vi "Autonomous Independent.vi"() -> ()   [LabVIEW 2014]
doc: "This VI is called when autonomous begins, and will automatically be terminated when autonomous ends. You can carry out timed or sensor driven robot movement independently without needing to return to the caller."
uses:
  Robot Global Data.vi
panel:
  in  "Close Claw Power 4":dbl=-0.8
  in  "Elevator Power 4":dbl=-0.8
  in  "Elevator to Tote1 drop distance 4":dbl=50.0
  in  "open claw pwr 3":dbl=0.8
  in  "Close Claw Power 3":dbl=-0.8
  in  "Elevator Power 3":dbl=-0.8
  in  "Elevator to Tote1 drop distance 3":dbl=50.0
  in  "Elevator to drop to tote distance 3":dbl=50.0
  in  "Drop elevator pwr 3":dbl=-0.8
  in  "Move up to tote 3":dbl=50.0
  out "reach Tote? 3":bool
  in  "Elevator to Raise distance":dbl=50.0
  in  "Raise Elevator Power 3":dbl=0.8
  out "Current Step 2":string
  in  "Move up to auto zone 2":dbl
  out "reach auto zone? 2":bool
  in  "Left Set Point 2":dbl=-65.0
  in  "Right Set Point 2":dbl=-35.0
  out "Make Turn? 2":bool
  in  "open claw pwr 2":dbl=0.8
  in  "Wait Time between each step 2":dbl=0.5
  in  "Elevator to drop to tote distance 2":dbl=50.0
  in  "Drop elevator pwr 2":dbl=-0.8
  in  "Move up to tote 2":dbl=50.0
  out "reach Tote? 2":bool
  in  "Elevator to Raise RC above tote 2":dbl=50.0
  in  "Raise Elevator Power 2":dbl=0.8
  in  "Close Claw Power 2":dbl=-0.8
  in  "Elevator Power 2":dbl=-0.8
  in  "Elevator to Tote1 drop distance 2":dbl=50.0
  in  "Claw Open Power 2":dbl=0.8
  in  "close claw pwr":dbl=-0.8
  in  "Drop elevator pwr":dbl=-0.8
  in  "Open Claw Power":dbl=0.8
  in  "Raise Elevator Power":dbl=0.8
  in  "Close Claw Power":dbl=-0.8
  in  "Claw Open Power":dbl=-0.8
  in  "Move up to auto zone":dbl
  out "reach auto zone?":bool
  out "Make Turn?":bool
  in  "Right Set Point":dbl=-35.0
  in  "Left Set Point":dbl=-65.0
  in  "Elevator to drop to tote distance":dbl=50.0
  in  "Elevator to Raise RC above tote":dbl=50.0
  in  "Elevator to RC drop distance":dbl=50.0
  out "Reach Distance?":bool
  in  "Elevator Power":dbl=-0.8
  in  "Wait Time between each step":dbl=0.5
  out "Current Step":string
  out "Right Encoder":dbl
  out "Left Encoder":dbl
  in  "Go Staight Distance":dbl=-50.0
  out "reach Tote?":bool
  in  "Move up to tote":dbl=50.0
  in  "Left Range":cluster{"output high":dbl, "output low":dbl}={"output high"=0.75, "output low"=-0.75} {"output low" format="%.2f"; "output high" format="%.2f"}
  in  "Left Gains":T1={"proportional gain (Kc)"=0.25, "integral time (Ti, min)"=0.0, "derivative time (Td, min)"=0.0} {"derivative time (Td, min)" format="%.3f"; "integral time (Ti, min)" format="%.3f"; "proportional gain (Kc)" format="%.3f"}
  in  "Right Gains":T1={"proportional gain (Kc)"=0.25, "integral time (Ti, min)"=0.0, "derivative time (Td, min)"=0.0} {"derivative time (Td, min)" format="%.3f"; "integral time (Ti, min)" format="%.3f"; "proportional gain (Kc)" format="%.3f"}
  in  "Right Range":cluster{"output high":dbl, "output low":dbl}={"output high"=0.75, "output low"=-0.75} {"output low" format="%.2f"; "output high" format="%.2f"}
  # "Auton Options"
  # "Be sure to right-click and choose Data Operations>>Make Current Value default if you want to save the array values with the VI"
  # "Stack RC on Tote and take them to auto zone"
  # "Stack RC on Tote and take them to auto zone"
  # "Open Claw"
  # "Open Claw"
  # "Drop Elevator to RC"
  # "Drop Elevator to Tote 1"
  # "Close Claw on RC"
  # "Close Claw on Tote 1"
  # "Raise RC above Tote"
  # "Raise Tote 1 above Tote 2"
  # "Approach Tote"
  # "Approach Tote 2"
  # "Lower tote 1 onto Tote 2"
  # "Open Claw"
  # "Open Claw"
  # "Drop Elevator to Tote"
  # "Close Claw on Tote"
  # "Drop Elevator to Tote 2"
  # "Turn Left"
  # "Close Claw on Tote 2"
  # "Go to Auto Zone"
  # "Raise Totes 1&2 above Tote 3"
  # "Approach Tote 3"
  # "Lower tote 1 & 2 onto Tote 3"
  # "Open Claw"
  # "Drop Elevator to Tote 3"
  # "Close Claw on Tote 3"
  # "Turn Right"
  # "Go to Auto Zone"
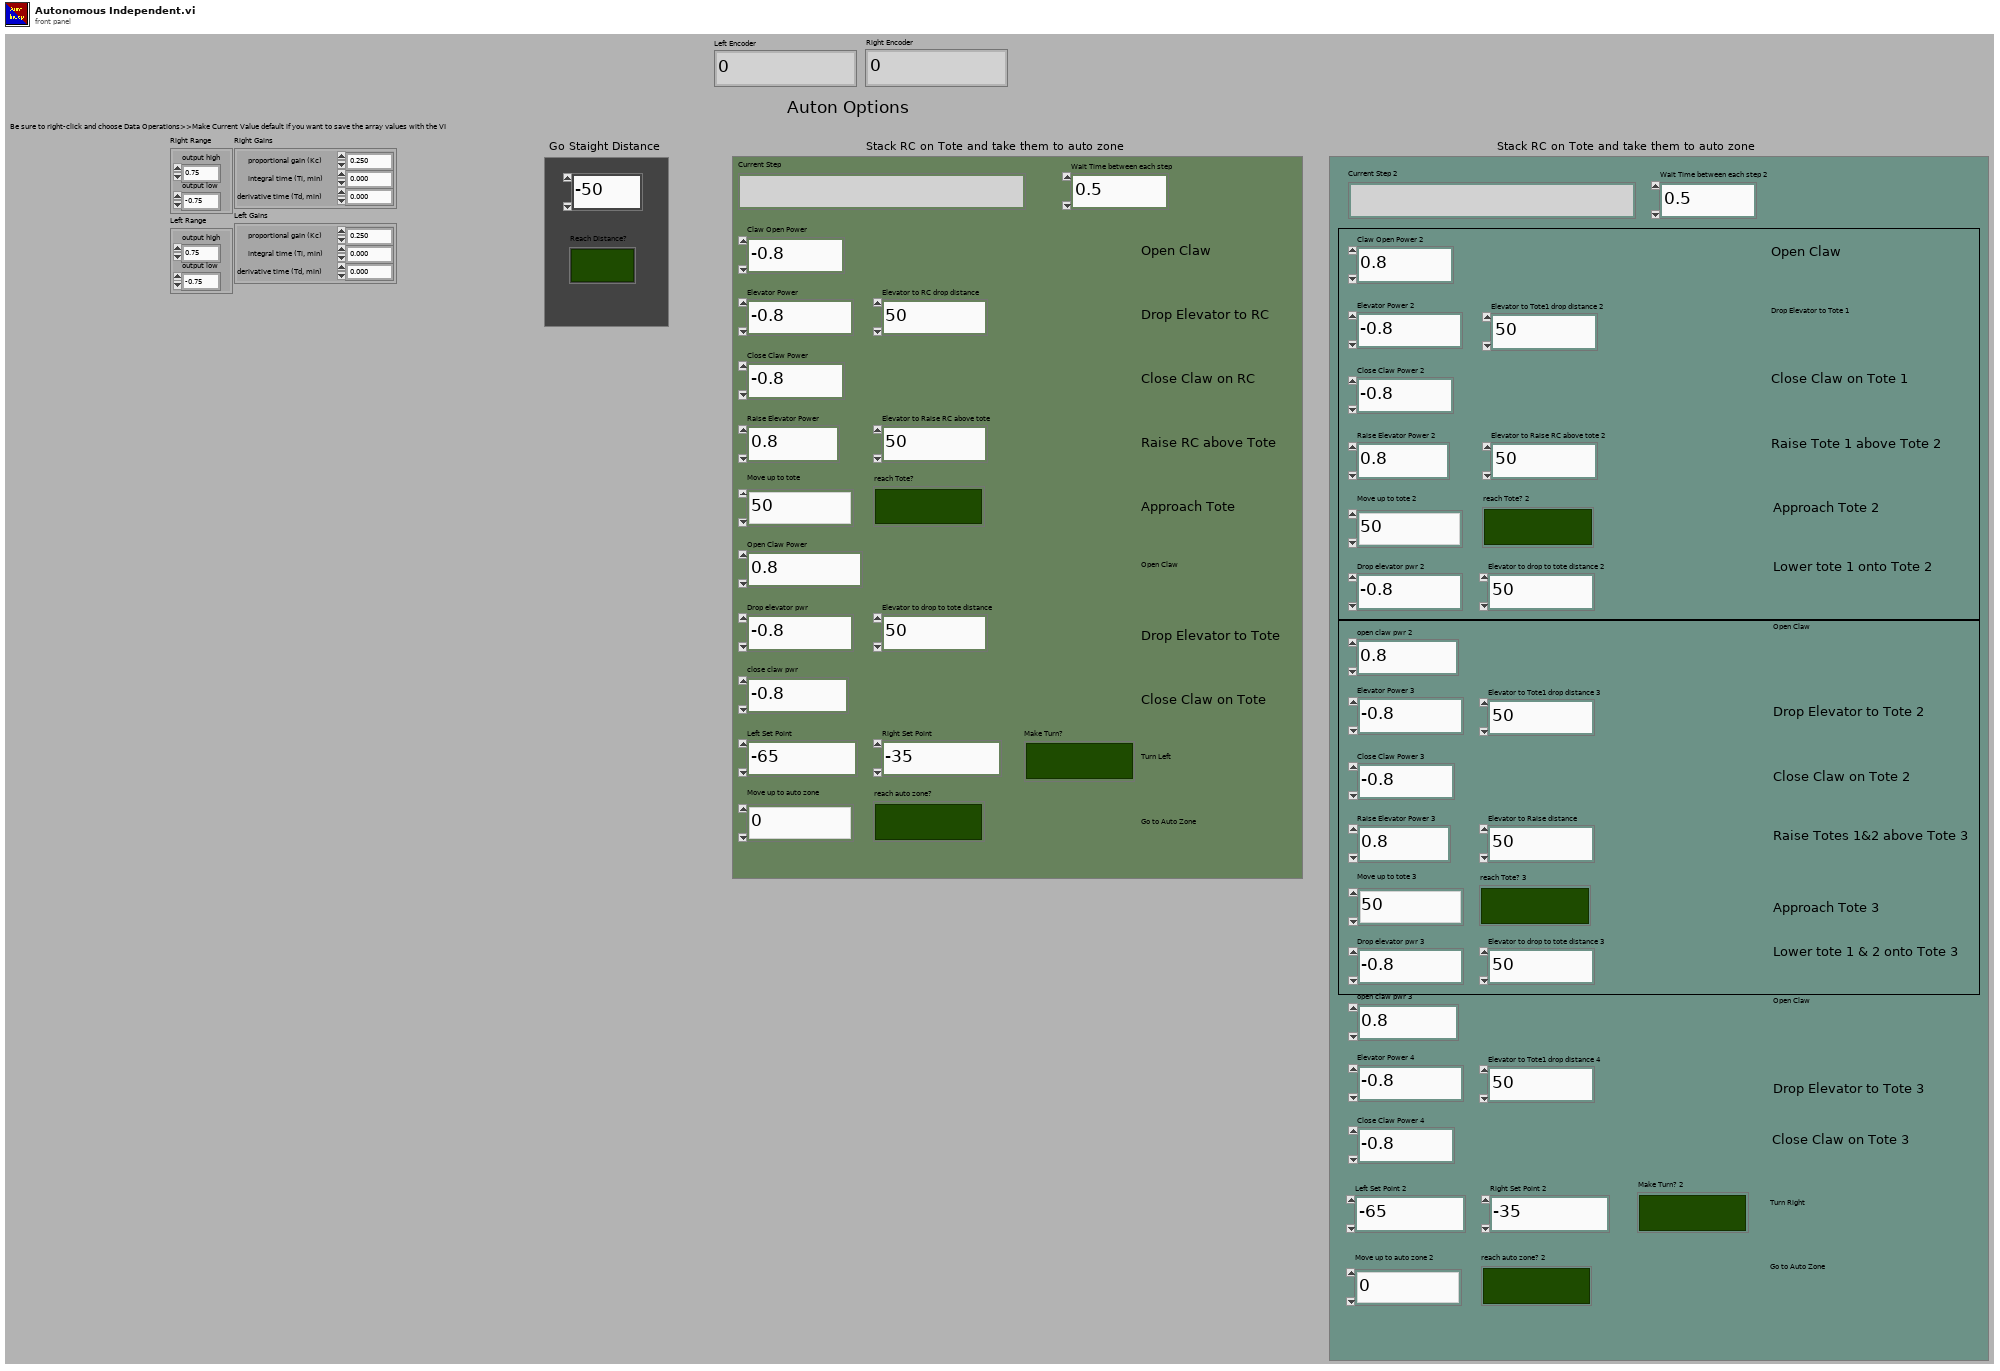
[diagram p1: front panel]
types:
  T1 = cluster{"proportional gain (Kc)":dbl, "integral time (Ti, min)":dbl, "derivative time (Td, min)":dbl}
  T2 = typedef "WPI_MotorControlDeviceRef.ctl" = cluster{"DeviceStatus":errorcluster, "Type":T3, "PWM":cluster{"Controller":T4, "PWM Channel":T5, "DeadBand":T6}, "CAN":cluster{"Device Number":u8, "Control Mode":T7, "Semaphore":T8, "Max Vout":dbl, "TalonSRX Control Mode":T9}, "Invert":bool, "TransformRef":T10, "InvTransformRef":T10}
  T3 = typedef "WPI_MotorControlType.ctl" = enum16{"PWM", "CAN", "CANTalonSRX"}
  T4 = typedef "FPGA_TypedefDigitalModule.ctl" = enum16{"Controller 1"}
  T5 = typedef "FPGA_DIOPWMChannel.ctl" = enum8{"PWM 0", "PWM 1", "PWM 2", "PWM 3", "PWM 4", "PWM 5", "PWM 6", "PWM 7", "PWM 8", "PWM 9", "PWM MXP 0", "PWM MXP 1", "PWM MXP 2", "PWM MXP 3", "PWM MXP 4", "PWM MXP 5", "PWM MXP 6", "PWM MXP 7", "PWM MXP 8", "PWM MXP 9", "Invalid"}
  T6 = typedef "WPI_PWMDeadband.ctl" = cluster{"Name":string, "maxPositivePwm":i32, "minPositivePwm":i32, "centerPwm":i32, "maxNegativePwm":i32, "minNegativePwm":i32, "angularRange":u16}
  T7 = typedef "WPI_CANJaguar_ControlMode.ctl" = enum8{"Percent VBus", "Current", "Speed", "Position", "Voltage"}
  T8 = typedef "Semaphore RefNum" = refnum<k1>
  T9 = typedef "WPI_CANTalonSRX_APIControlMode.ctl" = enum8{"Percent VBus", "Speed", "Position", "Slave", "Unchanged / Invalid"}
  T10 = typedef "WPI_PWMTransform_ConPane.ctl" = refnum<vi>
  T11 = typedef "WPI_EncoderDevRef.ctl" = cluster{"DevStatus":errorcluster, "EncoderIndex":T12, "CounterIndex":T13, "DistancePerCount":dbl, "Decoding Type":T14}
  T12 = typedef "FPGA_EncoderIdx.ctl" = enum8{"Enc 0", "Enc 1", "Enc 2", "Enc 3", "Enc 4", "Enc 5", "Enc 6", "Enc 7", "Invalid"}
  T13 = typedef "FPGA_CounterCtrSystemIndex.ctl" = enum8{"Ctr 0", "Ctr 1", "Ctr 2", "Ctr 3", "Ctr 4", "Ctr 5", "Ctr 6", "Ctr 7", "Invalid"}
  T14 = typedef "WPI_EncoderType.ctl" = enum16{"1x", "2x", "4x"}
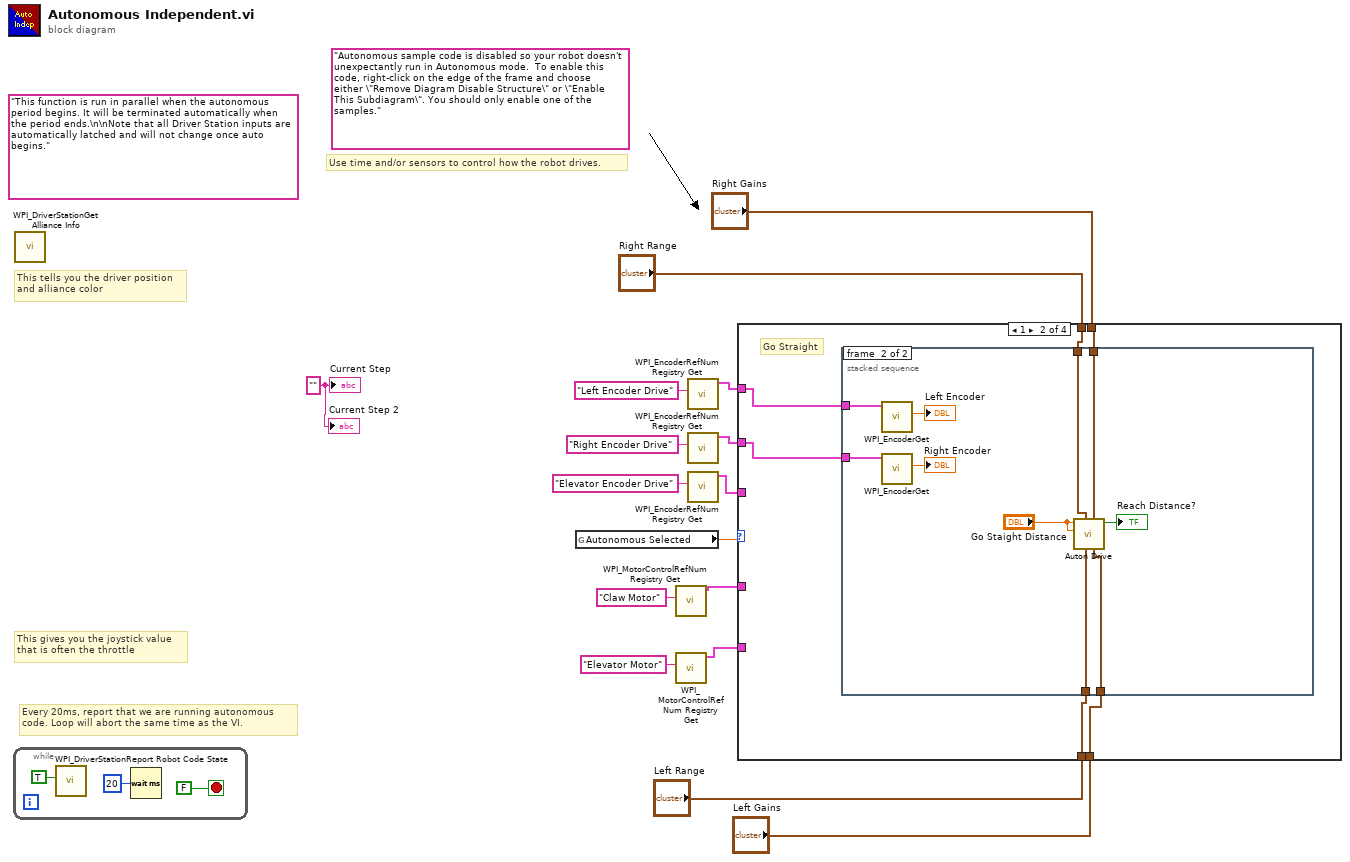
[diagram p0: block diagram]
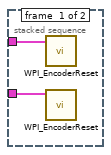
[diagram p3: hidden frame]
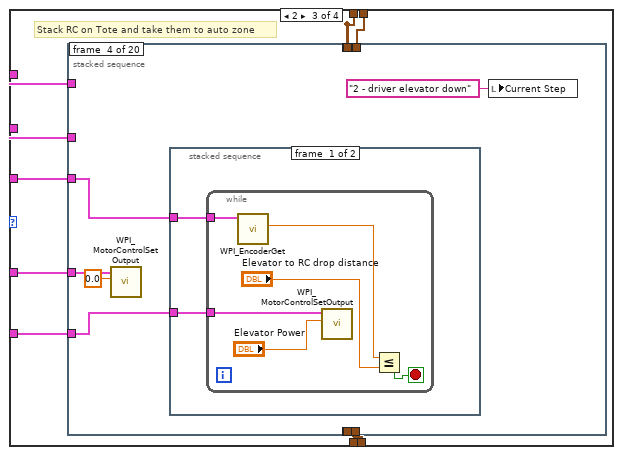
[diagram p4: hidden frame]
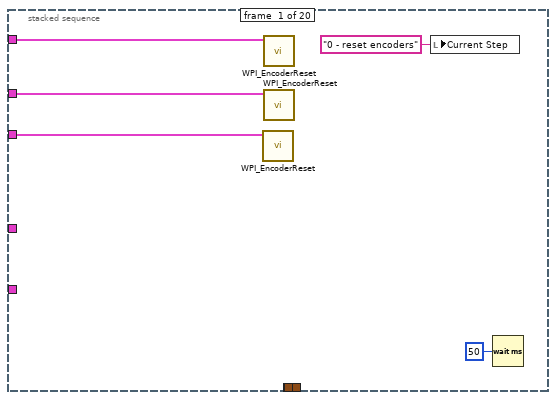
[diagram p5: hidden frame]
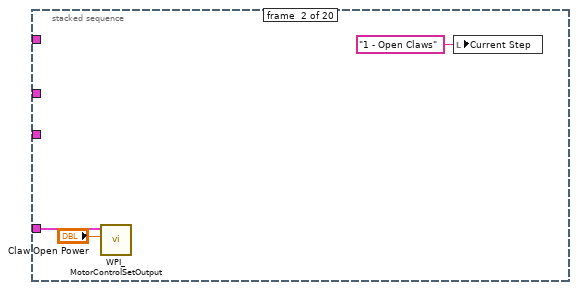
[diagram p6: hidden frame]
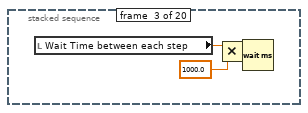
[diagram p7: hidden frame]
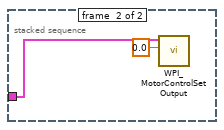
[diagram p8: hidden frame]
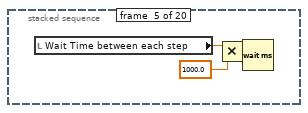
[diagram p9: hidden frame]
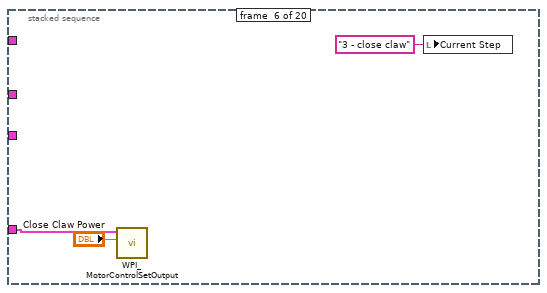
[diagram p10: hidden frame]
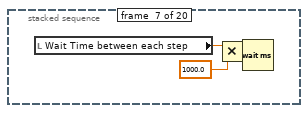
[diagram p11: hidden frame]
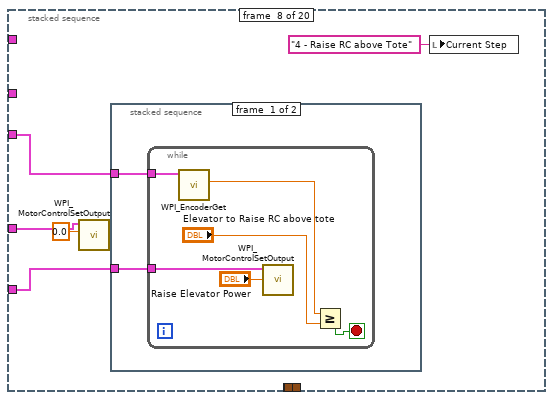
[diagram p12: hidden frame]
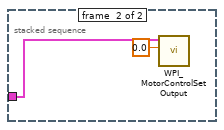
[diagram p13: hidden frame]
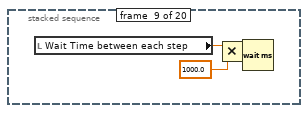
[diagram p14: hidden frame]
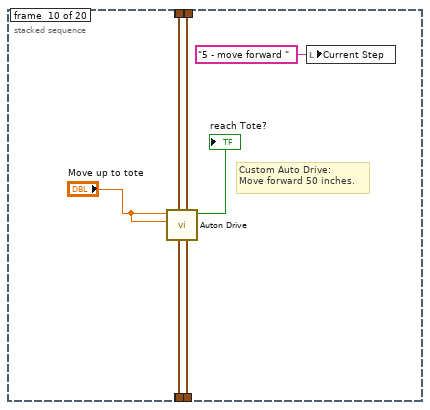
[diagram p15: hidden frame]
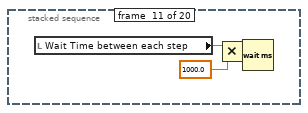
[diagram p16: hidden frame]
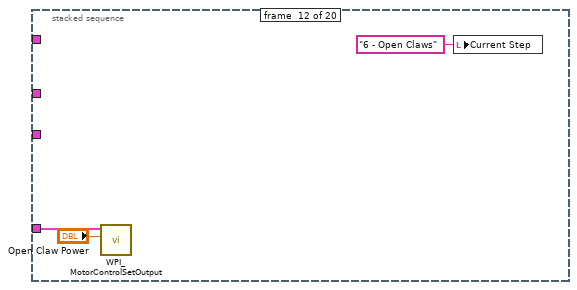
[diagram p17: hidden frame]
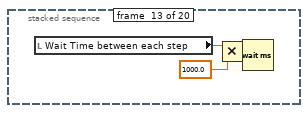
[diagram p18: hidden frame]
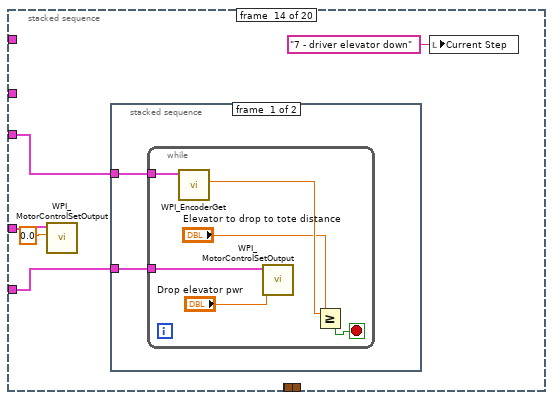
[diagram p19: hidden frame]
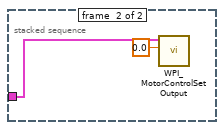
[diagram p20: hidden frame]
diagram:
  w1 = "" ("Current Step")
  (unwired) "Autonomous sample code is disabled so your robot doesn't unexpectantly run in Autonomous mode.  To enable this code, right-click on the edge of the frame and choose either \"Remove Diagram Disable Structure\" or \"Enable This Subdiagram\". You should only enable one of the samples."
  (unwired) "This function is run in parallel when the autonomous period begins. It will be terminated automatically when the period ends.\n\nNote that all Driver Station inputs are automatically latched and will not change once auto begins."
  # "Every 20ms, report that we are running autonomous\ncode. Loop will abort the same time as the VI."
  # "This gives you the joystick value\nthat is often the throttle"
  # "Use time and/or sensors to control how the robot drives."
  # "This tells you the driver position\nand alliance color"
  n1 = while {
    stop <- FALSE stop-if-true
    n2 = call <vilib>:"WPI_DriverStationReport Robot Code State.vi"("Autonomous"=TRUE) -> ()  [unwired: 10 in, 1 out]
    n3 = Wait (ms)(milliseconds to wait=u32 20) -> ()  [unwired: 1 out]
  }
  n4 = call <vilib>:"WPI_DriverStationGet Alliance Info.vi"() -> ()  [unwired: 12 out]
  n5 = global read "Robot Global Data.vi" "Autonomous Selected"() -> (w6:dbl)
  n6 = call <vilib>:"WPI_MotorControlRefNum Registry Get.vi"("refnum name"="Claw Motor") -> ("MotorControlDevRef"=w3:T2)  [unwired: 9 in, 1 out]
  n7 = call <vilib>:"WPI_MotorControlRefNum Registry Get.vi"("refnum name"="Elevator Motor") -> ("MotorControlDevRef"=w2:T2)  [unwired: 9 in, 1 out]
  n8 = call <vilib>:"WPI_EncoderRefNum Registry Get.vi"("refnum name"="Left Encoder Drive") -> ("EncoderDevRef"=w8:T11)  [unwired: 9 in, 1 out]
  n9 = call <vilib>:"WPI_EncoderRefNum Registry Get.vi"("refnum name"="Right Encoder Drive") -> ("EncoderDevRef"=w7:T11)  [unwired: 9 in, 1 out]
  n10 = call <vilib>:"WPI_EncoderRefNum Registry Get.vi"("refnum name"="Elevator Encoder Drive") -> ("EncoderDevRef"=w4:T11)  [unwired: 9 in, 1 out]
  n11 = case shown="1" w6 {
    tunnel: "Right Range" -> [_ w25 w46 w168]
    tunnel: "Right Gains" -> [_ w24 w45 w167]
    tunnel: "Left Range" -> [_ w23 w44 w166]
    tunnel: "Left Gains" -> [_ w22 w43 w165]
    tunnel: w8 -> [_ w21 w42 w164]
    tunnel: w7 -> [_ w20 w41 w163]
    tunnel: w4 -> [_ _ w40 w162]
    tunnel: w3 -> [_ _ w39 w161]
    tunnel: w2 -> [_ _ w38 w160]
    frame 0, Default {
      # "Do Nothing"
    }
    frame 1 {
      # "Go Straight"
      n12 = stacked-sequence {
        tunnel: w25 -> [_ w37]
        tunnel: w24 -> [_ w36]
        tunnel: w23 -> [_ w35]
        tunnel: w22 -> [_ w34]
        tunnel: w21 -> [w27 w32]
        tunnel: w20 -> [w26 w30]
        frame #0 {
          n13 = call <vilib>:"WPI_EncoderReset.vi"("EncoderDevRef"=w27) -> ()  [unwired: 9 in, 2 out]
          n14 = call <vilib>:"WPI_EncoderReset.vi"("EncoderDevRef"=w26) -> ()  [unwired: 9 in, 2 out]
        }
        frame #1 {
          n15 = call <vilib>:"WPI_EncoderGet.vi"("EncoderDevRef"=w32) -> ("Distance"=→"Left Encoder":dbl)  [unwired: 5 in, 5 out]
          n16 = call <vilib>:"WPI_EncoderGet.vi"("EncoderDevRef"=w30) -> ("Distance"=→"Right Encoder":dbl)  [unwired: 5 in, 5 out]
          n17 = call "Auton Drive.vi"("Left Gains"=w34, "Right Gains"=w36, "Left Range"=w35, "Right Range"=w37, "Right Set Point"="Go Staight Distance", "Left Set Point"="Go Staight Distance") -> ("At Destination?"=→"Reach Distance?":bool)  [unwired: 5 in]
        }
      }
    }
    frame 2 {
      # "Stack RC on Tote and take them to auto zone"
      n18 = stacked-sequence {
        tunnel: w42 -> [w51 _ _ _ _ _ _ _ _ _ _ _ _ _ _ _ _ _ _ _]
        tunnel: w41 -> [w50 _ _ _ _ _ _ _ _ _ _ _ _ _ _ _ _ _ _ _]
        tunnel: w46 -> [_ _ _ _ _ _ _ _ _ w106 _ _ _ _ _ _ _ _ _ w159]
        tunnel: w43 -> [_ _ _ _ _ _ _ _ _ w104 _ _ _ _ _ _ _ _ _ w157]
        tunnel: w44 -> [_ _ _ _ _ _ _ _ _ w103 _ _ _ _ _ _ _ _ _ w156]
        tunnel: w46 -> [_ _ _ _ _ _ _ _ _ _ _ _ _ _ _ _ _ w149 _ _]
        tunnel: w45 -> [_ _ _ _ _ _ _ _ _ w105 _ _ _ _ _ _ _ w148 _ w158]
        tunnel: w44 -> [_ _ _ _ _ _ _ _ _ _ _ _ _ _ _ _ _ w147 _ _]
        tunnel: w43 -> [_ _ _ _ _ _ _ _ _ _ _ _ _ _ _ _ _ w146 _ _]
        tunnel: w40 -> [w48 _ _ w60 _ _ _ w84 _ _ _ _ _ w118 _ _ _ _ _ _]
        tunnel: w39 -> [_ w53 _ w59 _ w77 _ w82 _ _ _ w111 _ w117 _ w136 _ w141 _ _]
        tunnel: w38 -> [_ _ _ w61 _ _ _ w85 _ _ _ _ _ w119 _ _ _ _ _ _]
        frame #0 {
          n19 = call <vilib>:"WPI_EncoderReset.vi"("EncoderDevRef"=w48) -> ()  [unwired: 9 in, 2 out]
          n20 = call <vilib>:"WPI_EncoderReset.vi"("EncoderDevRef"=w51) -> ()  [unwired: 9 in, 2 out]
          n21 = call <vilib>:"WPI_EncoderReset.vi"("EncoderDevRef"=w50) -> ()  [unwired: 9 in, 2 out]
          n22 = local write "Current Step"("0 - reset encoders" ("Current Step")) -> ()
          n23 = Wait (ms)(milliseconds to wait=u32 50) -> ()  [unwired: 1 out]
        }
        frame #1 {
          n24 = call <vilib>:"WPI_MotorControlSetOutput.vi"("Output"="Claw Open Power", "MotorControlDevRef"=w53) -> ()  [unwired: 7 in, 3 out]
          n25 = local write "Current Step"("1 - Open Claws" ("Current Step")) -> ()
        }
        frame #2 {
          n26 = local read "Wait Time between each step"() -> (w57:dbl)
          n27 = Multiply(x=w57, y=1000.0) -> (x*y=w56:dbl)
          n28 = Wait (ms)(milliseconds to wait=w56) -> ()  [unwired: 1 out]
        }
        frame #3 {
          n29 = call <vilib>:"WPI_MotorControlSetOutput.vi"("Output"=0.0, "MotorControlDevRef"=w59) -> ()  [unwired: 7 in, 3 out]
          n30 = stacked-sequence {
            tunnel: w61 -> [w64 w72]
            tunnel: w60 -> [w63 _]
            frame #0 {
              n31 = while {
                tunnel: w64 -> [w69]
                tunnel: w63 -> [w68]
                stop <- w67 stop-if-true
                n32 = call <vilib>:"WPI_EncoderGet.vi"("EncoderDevRef"=w68) -> ("Distance"=w66:dbl)  [unwired: 5 in, 5 out]
                n33 = call <vilib>:"WPI_MotorControlSetOutput.vi"("Output"="Elevator Power", "MotorControlDevRef"=w69) -> ()  [unwired: 7 in, 3 out]
                n34 = Less Or Equal?(x=w66, y="Elevator to RC drop distance") -> (x <= y?=w67:bool)
              }
            }
            frame #1 {
              n35 = call <vilib>:"WPI_MotorControlSetOutput.vi"("Output"=0.0, "MotorControlDevRef"=w72) -> ()  [unwired: 7 in, 3 out]
            }
          }
          n36 = local write "Current Step"("2 - driver elevator down" ("Current Step")) -> ()
        }
        frame #4 {
          n37 = local read "Wait Time between each step"() -> (w75:dbl)
          n38 = Multiply(x=w75, y=1000.0) -> (x*y=w74:dbl)
          n39 = Wait (ms)(milliseconds to wait=w74) -> ()  [unwired: 1 out]
        }
        frame #5 {
          n40 = call <vilib>:"WPI_MotorControlSetOutput.vi"("Output"="Close Claw Power", "MotorControlDevRef"=w77) -> ()  [unwired: 7 in, 3 out]
          n41 = local write "Current Step"("3 - close claw" ("Current Step")) -> ()
        }
        frame #6 {
          n42 = local read "Wait Time between each step"() -> (w81:dbl)
          n43 = Multiply(x=w81, y=1000.0) -> (x*y=w80:dbl)
          n44 = Wait (ms)(milliseconds to wait=w80) -> ()  [unwired: 1 out]
        }
        frame #7 {
          n45 = call <vilib>:"WPI_MotorControlSetOutput.vi"("Output"=0.0, "MotorControlDevRef"=w82) -> ()  [unwired: 7 in, 3 out]
          n46 = stacked-sequence {
            tunnel: w85 -> [w88 w96]
            tunnel: w84 -> [w87 _]
            frame #0 {
              n47 = while {
                tunnel: w88 -> [w94]
                tunnel: w87 -> [w93]
                stop <- w92 stop-if-true
                n48 = call <vilib>:"WPI_EncoderGet.vi"("EncoderDevRef"=w93) -> ("Distance"=w91:dbl)  [unwired: 5 in, 5 out]
                n49 = call <vilib>:"WPI_MotorControlSetOutput.vi"("Output"="Raise Elevator Power", "MotorControlDevRef"=w94) -> ()  [unwired: 7 in, 3 out]
                n50 = Greater Or Equal?(x=w91, y="Elevator to Raise RC above tote") -> (x >= y?=w92:bool)
              }
            }
            frame #1 {
              n51 = call <vilib>:"WPI_MotorControlSetOutput.vi"("Output"=0.0, "MotorControlDevRef"=w96) -> ()  [unwired: 7 in, 3 out]
            }
          }
          n52 = local write "Current Step"("4 - Raise RC above Tote" ("Current Step")) -> ()
        }
        frame #8 {
          n53 = local read "Wait Time between each step"() -> (w99:dbl)
          n54 = Multiply(x=w99, y=1000.0) -> (x*y=w98:dbl)
          n55 = Wait (ms)(milliseconds to wait=w98) -> ()  [unwired: 1 out]
        }
        frame #9 {
          # "Custom Auto Drive:\nMove forward 50 inches."
          n56 = call "Auton Drive.vi"("Left Gains"=w104, "Right Gains"=w105, "Left Range"=w103, "Right Range"=w106, "Right Set Point"="Move up to tote", "Left Set Point"="Move up to tote") -> ("At Destination?"=→"reach Tote?":bool)  [unwired: 5 in]
          n57 = local write "Current Step"("5 - move forward " ("Current Step")) -> ()
        }
        frame #10 {
          n58 = local read "Wait Time between each step"() -> (w109:dbl)
          n59 = Multiply(x=w109, y=1000.0) -> (x*y=w108:dbl)
          n60 = Wait (ms)(milliseconds to wait=w108) -> ()  [unwired: 1 out]
        }
        frame #11 {
          n61 = call <vilib>:"WPI_MotorControlSetOutput.vi"("Output"="Open Claw Power", "MotorControlDevRef"=w111) -> ()  [unwired: 7 in, 3 out]
          n62 = local write "Current Step"("6 - Open Claws" ("Current Step")) -> ()
        }
        frame #12 {
          n63 = local read "Wait Time between each step"() -> (w115:dbl)
          n64 = Multiply(x=w115, y=1000.0) -> (x*y=w114:dbl)
          n65 = Wait (ms)(milliseconds to wait=w114) -> ()  [unwired: 1 out]
        }
        frame #13 {
          n66 = call <vilib>:"WPI_MotorControlSetOutput.vi"("Output"=0.0, "MotorControlDevRef"=w117) -> ()  [unwired: 7 in, 3 out]
          n67 = stacked-sequence {
            tunnel: w119 -> [w122 w130]
            tunnel: w118 -> [w121 _]
            frame #0 {
              n68 = while {
                tunnel: w122 -> [w128]
                tunnel: w121 -> [w127]
                stop <- w126 stop-if-true
                n69 = call <vilib>:"WPI_EncoderGet.vi"("EncoderDevRef"=w127) -> ("Distance"=w125:dbl)  [unwired: 5 in, 5 out]
                n70 = call <vilib>:"WPI_MotorControlSetOutput.vi"("Output"="Drop elevator pwr", "MotorControlDevRef"=w128) -> ()  [unwired: 7 in, 3 out]
                n71 = Greater Or Equal?(x=w125, y="Elevator to drop to tote distance") -> (x >= y?=w126:bool)
              }
            }
            frame #1 {
              n72 = call <vilib>:"WPI_MotorControlSetOutput.vi"("Output"=0.0, "MotorControlDevRef"=w130) -> ()  [unwired: 7 in, 3 out]
            }
          }
          n73 = local write "Current Step"("7 - driver elevator down" ("Current Step")) -> ()
        }
        frame #14 {
          n74 = Multiply(x="Wait Time between each step", y=1000.0) -> (x*y=w133:dbl)
          n75 = Wait (ms)(milliseconds to wait=w133) -> ()  [unwired: 1 out]
        }
        frame #15 {
          n76 = call <vilib>:"WPI_MotorControlSetOutput.vi"("Output"="close claw pwr", "MotorControlDevRef"=w136) -> ()  [unwired: 7 in, 3 out]
          n77 = local write "Current Step"("8 - closer claw on tote" ("Current Step")) -> ()
        }
        frame #16 {
          n78 = local read "Wait Time between each step"() -> (w139:dbl)
          n79 = Multiply(x=w139, y=1000.0) -> (x*y=w138:dbl)
          n80 = Wait (ms)(milliseconds to wait=w138) -> ()  [unwired: 1 out]
        }
        frame #17 {
          # "Turn 10 inches (In wheel rotations) to the right."
          n81 = call <vilib>:"WPI_MotorControlSetOutput.vi"("Output"=0.0, "MotorControlDevRef"=w141) -> ()  [unwired: 7 in, 3 out]
          n82 = call "Auton Drive.vi"("Left Gains"=w146, "Right Gains"=w148, "Left Range"=w147, "Right Range"=w149, "Right Set Point"="Right Set Point", "Left Set Point"="Left Set Point") -> ("At Destination?"=→"Make Turn?":bool)  [unwired: 5 in]
          n83 = local write "Current Step"("9 - Turn Left" ("Current Step")) -> ()
        }
        frame #18 {
          n84 = local read "Wait Time between each step"() -> (w152:dbl)
          n85 = Multiply(x=w152, y=1000.0) -> (x*y=w151:dbl)
          n86 = Wait (ms)(milliseconds to wait=w151) -> ()  [unwired: 1 out]
        }
        frame #19 {
          # "Custom Auto Drive:\nMove forward 50 inches."
          n87 = call "Auton Drive.vi"("Left Gains"=w157, "Right Gains"=w158, "Left Range"=w156, "Right Range"=w159, "Right Set Point"="Move up to auto zone", "Left Set Point"="Move up to auto zone") -> ("At Destination?"=→"reach auto zone?":bool)  [unwired: 5 in]
          n88 = local write "Current Step"("10 - move to auto zone" ("Current Step")) -> ()
        }
      }
    }
    frame 3 {
      # "Stack RC on Tote and take them to auto zone"
      n89 = stacked-sequence {
        tunnel: w164 -> [w173 _ _ _ _ _ _ _ _ _ _ _ _ _ _ _ _ _ _ _ _ _ _ _ _ _ _ _ _ _ _ _ _ _]
        tunnel: w163 -> [w172 _ _ _ _ _ _ _ _ _ _ _ _ _ _ _ _ _ _ _ _ _ _ _ _ _ _ _ _ _ _ _ _ _]
        tunnel: w168 -> [_ _ _ _ _ _ _ _ _ w228 _ _ _ _ _ _ _ _ _ _ _ w304 _ _ _ _ _ _ _ _ _ _ _ w375]
        tunnel: w165 -> [_ _ _ _ _ _ _ _ _ w226 _ _ _ _ _ _ _ _ _ _ _ w302 _ _ _ _ _ _ _ _ _ _ _ w373]
        tunnel: w166 -> [_ _ _ _ _ _ _ _ _ w225 _ _ _ _ _ _ _ _ _ _ _ w301 _ _ _ _ _ _ _ _ _ _ _ w372]
        tunnel: w168 -> [_ _ _ _ _ _ _ _ _ _ _ _ _ _ _ _ _ _ _ _ _ _ _ _ _ _ _ _ _ _ _ w365 _ _]
        tunnel: w167 -> [_ _ _ _ _ _ _ _ _ w227 _ _ _ _ _ _ _ _ _ _ _ w303 _ _ _ _ _ _ _ _ _ w364 _ w374]
        tunnel: w166 -> [_ _ _ _ _ _ _ _ _ _ _ _ _ _ _ _ _ _ _ _ _ _ _ _ _ _ _ _ _ _ _ w363 _ _]
        tunnel: w165 -> [_ _ _ _ _ _ _ _ _ _ _ _ _ _ _ _ _ _ _ _ _ _ _ _ _ _ _ _ _ _ _ w362 _ _]
        tunnel: w162 -> [w170 _ _ w182 _ _ _ w206 _ _ _ w234 _ _ _ w258 _ _ _ w282 _ _ _ w310 _ _ _ w334 _ _ _ _ _ _]
        tunnel: w161 -> [_ w175 _ w181 _ w199 _ w204 _ _ _ w233 _ w252 _ w257 _ w275 _ w280 _ _ _ w309 _ w328 _ w333 _ w351 _ w357 _ _]
        tunnel: w160 -> [_ _ _ w183 _ _ _ w207 _ _ _ w235 _ _ _ w259 _ _ _ w283 _ _ _ w311 _ _ _ w335 _ _ _ _ _ _]
        frame #0 {
          n90 = call <vilib>:"WPI_EncoderReset.vi"("EncoderDevRef"=w170) -> ()  [unwired: 9 in, 2 out]
          n91 = call <vilib>:"WPI_EncoderReset.vi"("EncoderDevRef"=w173) -> ()  [unwired: 9 in, 2 out]
          n92 = call <vilib>:"WPI_EncoderReset.vi"("EncoderDevRef"=w172) -> ()  [unwired: 9 in, 2 out]
          n93 = local write "Current Step 2"("0 - reset encoders" ("Current Step")) -> ()
          n94 = Wait (ms)(milliseconds to wait=u32 50) -> ()  [unwired: 1 out]
        }
        frame #1 {
          n95 = call <vilib>:"WPI_MotorControlSetOutput.vi"("Output"="Claw Open Power 2", "MotorControlDevRef"=w175) -> ()  [unwired: 7 in, 3 out]
          n96 = local write "Current Step 2"("1 - Open Claws" ("Current Step")) -> ()
        }
        frame #2 {
          n97 = local read "Wait Time between each step 2"() -> (w179:dbl)
          n98 = Multiply(x=w179, y=1000.0) -> (x*y=w178:dbl)
          n99 = Wait (ms)(milliseconds to wait=w178) -> ()  [unwired: 1 out]
        }
        frame #3 {
          n100 = call <vilib>:"WPI_MotorControlSetOutput.vi"("Output"=0.0, "MotorControlDevRef"=w181) -> ()  [unwired: 7 in, 3 out]
          n101 = stacked-sequence {
            tunnel: w183 -> [w186 w194]
            tunnel: w182 -> [w185 _]
            frame #0 {
              n102 = while {
                tunnel: w186 -> [w191]
                tunnel: w185 -> [w190]
                stop <- w189 stop-if-true
                n103 = call <vilib>:"WPI_EncoderGet.vi"("EncoderDevRef"=w190) -> ("Distance"=w188:dbl)  [unwired: 5 in, 5 out]
                n104 = call <vilib>:"WPI_MotorControlSetOutput.vi"("Output"="Elevator Power 2", "MotorControlDevRef"=w191) -> ()  [unwired: 7 in, 3 out]
                n105 = Less Or Equal?(x=w188, y="Elevator to Tote1 drop distance 2") -> (x <= y?=w189:bool)
              }
            }
            frame #1 {
              n106 = call <vilib>:"WPI_MotorControlSetOutput.vi"("Output"=0.0, "MotorControlDevRef"=w194) -> ()  [unwired: 7 in, 3 out]
            }
          }
          n107 = local write "Current Step 2"("2 - driver elevator down to tote 1" ("Current Step")) -> ()
        }
        frame #4 {
          n108 = local read "Wait Time between each step 2"() -> (w197:dbl)
          n109 = Multiply(x=w197, y=1000.0) -> (x*y=w196:dbl)
          n110 = Wait (ms)(milliseconds to wait=w196) -> ()  [unwired: 1 out]
        }
        frame #5 {
          n111 = call <vilib>:"WPI_MotorControlSetOutput.vi"("Output"="Close Claw Power 2", "MotorControlDevRef"=w199) -> ()  [unwired: 7 in, 3 out]
          n112 = local write "Current Step 2"("3 - close claw" ("Current Step")) -> ()
        }
        frame #6 {
          n113 = local read "Wait Time between each step 2"() -> (w203:dbl)
          n114 = Multiply(x=w203, y=1000.0) -> (x*y=w202:dbl)
          n115 = Wait (ms)(milliseconds to wait=w202) -> ()  [unwired: 1 out]
        }
        frame #7 {
          n116 = call <vilib>:"WPI_MotorControlSetOutput.vi"("Output"=0.0, "MotorControlDevRef"=w204) -> ()  [unwired: 7 in, 3 out]
          n117 = stacked-sequence {
            tunnel: w207 -> [w210 w218]
            tunnel: w206 -> [w209 _]
            frame #0 {
              n118 = while {
                tunnel: w210 -> [w216]
                tunnel: w209 -> [w215]
                stop <- w214 stop-if-true
                n119 = call <vilib>:"WPI_EncoderGet.vi"("EncoderDevRef"=w215) -> ("Distance"=w213:dbl)  [unwired: 5 in, 5 out]
                n120 = call <vilib>:"WPI_MotorControlSetOutput.vi"("Output"="Raise Elevator Power 2", "MotorControlDevRef"=w216) -> ()  [unwired: 7 in, 3 out]
                n121 = Greater Or Equal?(x=w213, y="Elevator to Raise RC above tote 2") -> (x >= y?=w214:bool)
              }
            }
            frame #1 {
              n122 = call <vilib>:"WPI_MotorControlSetOutput.vi"("Output"=0.0, "MotorControlDevRef"=w218) -> ()  [unwired: 7 in, 3 out]
            }
          }
          n123 = local write "Current Step 2"("4 - Raise tote1 above Tote2" ("Current Step")) -> ()
        }
        frame #8 {
          n124 = local read "Wait Time between each step 2"() -> (w221:dbl)
          n125 = Multiply(x=w221, y=1000.0) -> (x*y=w220:dbl)
          n126 = Wait (ms)(milliseconds to wait=w220) -> ()  [unwired: 1 out]
        }
        frame #9 {
          # "Custom Auto Drive:\nMove forward 50 inches."
          n127 = call "Auton Drive.vi"("Left Gains"=w226, "Right Gains"=w227, "Left Range"=w225, "Right Range"=w228, "Right Set Point"="Move up to tote 2", "Left Set Point"="Move up to tote 2") -> ("At Destination?"=→"reach Tote? 2":bool)  [unwired: 5 in]
          n128 = local write "Current Step 2"("5 - move to tote 2 " ("Current Step")) -> ()
        }
        frame #10 {
          n129 = local read "Wait Time between each step 2"() -> (w231:dbl)
          n130 = Multiply(x=w231, y=1000.0) -> (x*y=w230:dbl)
          n131 = Wait (ms)(milliseconds to wait=w230) -> ()  [unwired: 1 out]
        }
        frame #11 {
          n132 = call <vilib>:"WPI_MotorControlSetOutput.vi"("Output"=0.0, "MotorControlDevRef"=w233) -> ()  [unwired: 7 in, 3 out]
          n133 = stacked-sequence {
            tunnel: w235 -> [w238 w246]
            tunnel: w234 -> [w237 _]
            frame #0 {
              n134 = while {
                tunnel: w238 -> [w244]
                tunnel: w237 -> [w243]
                stop <- w242 stop-if-true
                n135 = call <vilib>:"WPI_EncoderGet.vi"("EncoderDevRef"=w243) -> ("Distance"=w241:dbl)  [unwired: 5 in, 5 out]
                n136 = call <vilib>:"WPI_MotorControlSetOutput.vi"("Output"="Drop elevator pwr 2", "MotorControlDevRef"=w244) -> ()  [unwired: 7 in, 3 out]
                n137 = Greater Or Equal?(x=w241, y="Elevator to drop to tote distance 2") -> (x >= y?=w242:bool)
              }
            }
            frame #1 {
              n138 = call <vilib>:"WPI_MotorControlSetOutput.vi"("Output"=0.0, "MotorControlDevRef"=w246) -> ()  [unwired: 7 in, 3 out]
            }
          }
          n139 = local write "Current Step 2"("6 -elevator down on tote2" ("Current Step")) -> ()
        }
        frame #12 {
          n140 = Multiply(x="Wait Time between each step 2", y=1000.0) -> (x*y=w249:dbl)
          n141 = Wait (ms)(milliseconds to wait=w249) -> ()  [unwired: 1 out]
        }
        frame #13 {
          n142 = call <vilib>:"WPI_MotorControlSetOutput.vi"("Output"="open claw pwr 2", "MotorControlDevRef"=w252) -> ()  [unwired: 7 in, 3 out]
          n143 = local write "Current Step 2"("7 - open claw on tote1" ("Current Step")) -> ()
        }
        frame #14 {
          n144 = local read "Wait Time between each step 2"() -> (w255:dbl)
          n145 = Multiply(x=w255, y=1000.0) -> (x*y=w254:dbl)
          n146 = Wait (ms)(milliseconds to wait=w254) -> ()  [unwired: 1 out]
        }
        frame #15 {
          n147 = call <vilib>:"WPI_MotorControlSetOutput.vi"("Output"=0.0, "MotorControlDevRef"=w257) -> ()  [unwired: 7 in, 3 out]
          n148 = stacked-sequence {
            tunnel: w259 -> [w262 w270]
            tunnel: w258 -> [w261 _]
            frame #0 {
              n149 = while {
                tunnel: w262 -> [w267]
                tunnel: w261 -> [w266]
                stop <- w265 stop-if-true
                n150 = call <vilib>:"WPI_EncoderGet.vi"("EncoderDevRef"=w266) -> ("Distance"=w264:dbl)  [unwired: 5 in, 5 out]
                n151 = call <vilib>:"WPI_MotorControlSetOutput.vi"("Output"="Elevator Power 3", "MotorControlDevRef"=w267) -> ()  [unwired: 7 in, 3 out]
                n152 = Less Or Equal?(x=w264, y="Elevator to Tote1 drop distance 3") -> (x <= y?=w265:bool)
              }
            }
            frame #1 {
              n153 = call <vilib>:"WPI_MotorControlSetOutput.vi"("Output"=0.0, "MotorControlDevRef"=w270) -> ()  [unwired: 7 in, 3 out]
            }
          }
          n154 = local write "Current Step 2"("8 - elevator down to tote2" ("Current Step")) -> ()
        }
        frame #16 {
          n155 = local read "Wait Time between each step 2"() -> (w273:dbl)
          n156 = Multiply(x=w273, y=1000.0) -> (x*y=w272:dbl)
          n157 = Wait (ms)(milliseconds to wait=w272) -> ()  [unwired: 1 out]
        }
        frame #17 {
          n158 = call <vilib>:"WPI_MotorControlSetOutput.vi"("Output"="Close Claw Power 3", "MotorControlDevRef"=w275) -> ()  [unwired: 7 in, 3 out]
          n159 = local write "Current Step 2"("9 - close claw on tote2" ("Current Step")) -> ()
        }
        frame #18 {
          n160 = local read "Wait Time between each step 2"() -> (w279:dbl)
          n161 = Multiply(x=w279, y=1000.0) -> (x*y=w278:dbl)
          n162 = Wait (ms)(milliseconds to wait=w278) -> ()  [unwired: 1 out]
        }
        frame #19 {
          n163 = call <vilib>:"WPI_MotorControlSetOutput.vi"("Output"=0.0, "MotorControlDevRef"=w280) -> ()  [unwired: 7 in, 3 out]
          n164 = stacked-sequence {
            tunnel: w283 -> [w286 w294]
            tunnel: w282 -> [w285 _]
            frame #0 {
              n165 = while {
                tunnel: w286 -> [w292]
                tunnel: w285 -> [w291]
                stop <- w290 stop-if-true
                n166 = call <vilib>:"WPI_EncoderGet.vi"("EncoderDevRef"=w291) -> ("Distance"=w289:dbl)  [unwired: 5 in, 5 out]
                n167 = call <vilib>:"WPI_MotorControlSetOutput.vi"("Output"="Raise Elevator Power 3", "MotorControlDevRef"=w292) -> ()  [unwired: 7 in, 3 out]
                n168 = Greater Or Equal?(x=w289, y="Elevator to Raise distance") -> (x >= y?=w290:bool)
              }
            }
            frame #1 {
              n169 = call <vilib>:"WPI_MotorControlSetOutput.vi"("Output"=0.0, "MotorControlDevRef"=w294) -> ()  [unwired: 7 in, 3 out]
            }
          }
          n170 = local write "Current Step 2"("10 - Raise totes 1 & 2 above Tote3" ("Current Step")) -> ()
        }
        frame #20 {
          n171 = local read "Wait Time between each step 2"() -> (w297:dbl)
          n172 = Multiply(x=w297, y=1000.0) -> (x*y=w296:dbl)
          n173 = Wait (ms)(milliseconds to wait=w296) -> ()  [unwired: 1 out]
        }
        frame #21 {
          # "Custom Auto Drive:\nMove forward 50 inches."
          n174 = call "Auton Drive.vi"("Left Gains"=w302, "Right Gains"=w303, "Left Range"=w301, "Right Range"=w304, "Right Set Point"="Move up to tote 3", "Left Set Point"="Move up to tote 3") -> ("At Destination?"=→"reach Tote? 3":bool)  [unwired: 5 in]
          n175 = local write "Current Step 2"("11 - move to tote3" ("Current Step")) -> ()
        }
        frame #22 {
          n176 = local read "Wait Time between each step 2"() -> (w307:dbl)
          n177 = Multiply(x=w307, y=1000.0) -> (x*y=w306:dbl)
          n178 = Wait (ms)(milliseconds to wait=w306) -> ()  [unwired: 1 out]
        }
        frame #23 {
          n179 = call <vilib>:"WPI_MotorControlSetOutput.vi"("Output"=0.0, "MotorControlDevRef"=w309) -> ()  [unwired: 7 in, 3 out]
          n180 = stacked-sequence {
            tunnel: w311 -> [w314 w322]
            tunnel: w310 -> [w313 _]
            frame #0 {
              n181 = while {
                tunnel: w314 -> [w320]
                tunnel: w313 -> [w319]
                stop <- w318 stop-if-true
                n182 = call <vilib>:"WPI_EncoderGet.vi"("EncoderDevRef"=w319) -> ("Distance"=w317:dbl)  [unwired: 5 in, 5 out]
                n183 = call <vilib>:"WPI_MotorControlSetOutput.vi"("Output"="Drop elevator pwr 3", "MotorControlDevRef"=w320) -> ()  [unwired: 7 in, 3 out]
                n184 = Greater Or Equal?(x=w317, y="Elevator to drop to tote distance 3") -> (x >= y?=w318:bool)
              }
            }
            frame #1 {
              n185 = call <vilib>:"WPI_MotorControlSetOutput.vi"("Output"=0.0, "MotorControlDevRef"=w322) -> ()  [unwired: 7 in, 3 out]
            }
          }
          n186 = local write "Current Step 2"("12 -elevator down onto tote3" ("Current Step")) -> ()
        }
        frame #24 {
          n187 = local read "Wait Time between each step 2"() -> (w325:dbl)
          n188 = Multiply(x=w325, y=1000.0) -> (x*y=w324:dbl)
          n189 = Wait (ms)(milliseconds to wait=w324) -> ()  [unwired: 1 out]
        }
        frame #25 {
          n190 = call <vilib>:"WPI_MotorControlSetOutput.vi"("Output"="open claw pwr 3", "MotorControlDevRef"=w328) -> ()  [unwired: 7 in, 3 out]
          n191 = local write "Current Step 2"("13 - open claw on tote2" ("Current Step")) -> ()
        }
        frame #26 {
          n192 = local read "Wait Time between each step 2"() -> (w329:dbl)
          n193 = Multiply(x=w329, y=1000.0) -> (x*y=w331:dbl)
          n194 = Wait (ms)(milliseconds to wait=w331) -> ()  [unwired: 1 out]
        }
        frame #27 {
          n195 = call <vilib>:"WPI_MotorControlSetOutput.vi"("Output"=0.0, "MotorControlDevRef"=w333) -> ()  [unwired: 7 in, 3 out]
          n196 = stacked-sequence {
            tunnel: w335 -> [w338 w346]
            tunnel: w334 -> [w337 _]
            frame #0 {
              n197 = while {
                tunnel: w338 -> [w343]
                tunnel: w337 -> [w342]
                stop <- w341 stop-if-true
                n198 = call <vilib>:"WPI_EncoderGet.vi"("EncoderDevRef"=w342) -> ("Distance"=w340:dbl)  [unwired: 5 in, 5 out]
                n199 = call <vilib>:"WPI_MotorControlSetOutput.vi"("Output"="Elevator Power 4", "MotorControlDevRef"=w343) -> ()  [unwired: 7 in, 3 out]
                n200 = Less Or Equal?(x=w340, y="Elevator to Tote1 drop distance 4") -> (x <= y?=w341:bool)
              }
            }
            frame #1 {
              n201 = call <vilib>:"WPI_MotorControlSetOutput.vi"("Output"=0.0, "MotorControlDevRef"=w346) -> ()  [unwired: 7 in, 3 out]
            }
          }
          n202 = local write "Current Step 2"("14 -elevator down to tote 3" ("Current Step")) -> ()
        }
        frame #28 {
          n203 = local read "Wait Time between each step 2"() -> (w347:dbl)
          n204 = Multiply(x=w347, y=1000.0) -> (x*y=w349:dbl)
          n205 = Wait (ms)(milliseconds to wait=w349) -> ()  [unwired: 1 out]
        }
        frame #29 {
          n206 = call <vilib>:"WPI_MotorControlSetOutput.vi"("Output"="Close Claw Power 4", "MotorControlDevRef"=w351) -> ()  [unwired: 7 in, 3 out]
          n207 = local write "Current Step 2"("9 - close claw on tote3" ("Current Step")) -> ()
        }
        frame #30 {
          n208 = local read "Wait Time between each step 2"() -> (w355:dbl)
          n209 = Multiply(x=w355, y=1000.0) -> (x*y=w354:dbl)
          n210 = Wait (ms)(milliseconds to wait=w354) -> ()  [unwired: 1 out]
        }
        frame #31 {
          # "Turn 10 inches (In wheel rotations) to the right."
          n211 = call <vilib>:"WPI_MotorControlSetOutput.vi"("Output"=0.0, "MotorControlDevRef"=w357) -> ()  [unwired: 7 in, 3 out]
          n212 = call "Auton Drive.vi"("Left Gains"=w362, "Right Gains"=w364, "Left Range"=w363, "Right Range"=w365, "Right Set Point"="Right Set Point 2", "Left Set Point"="Left Set Point 2") -> ("At Destination?"=→"Make Turn? 2":bool)  [unwired: 5 in]
          n213 = local write "Current Step 2"("15 - Turn Right" ("Current Step")) -> ()
        }
        frame #32 {
          n214 = local read "Wait Time between each step 2"() -> (w368:dbl)
          n215 = Multiply(x=w368, y=1000.0) -> (x*y=w367:dbl)
          n216 = Wait (ms)(milliseconds to wait=w367) -> ()  [unwired: 1 out]
        }
        frame #33 {
          # "Custom Auto Drive:\nMove forward 50 inches."
          n217 = call "Auton Drive.vi"("Left Gains"=w373, "Right Gains"=w374, "Left Range"=w372, "Right Range"=w375, "Right Set Point"="Move up to auto zone 2", "Left Set Point"="Move up to auto zone 2") -> ("At Destination?"=→"reach auto zone? 2":bool)  [unwired: 5 in]
          n218 = local write "Current Step 2"("16 - move to auto zone" ("Current Step")) -> ()
        }
      }
    }
  }
  "Current Step" <- w1
  "Current Step 2" <- w1
